vi "Error Converter (ErrCode or Status).vi"(8 "error in (no error)":errorcluster, 11 "error code":i32) -> (0 "error out":errorcluster)   [LabVIEW 2020, in "sqlite3.lvlib"]
uses:
  sqlite3.lvlib
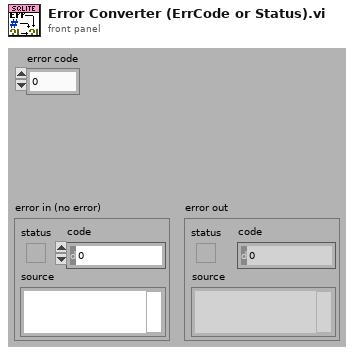
[diagram p1: front panel]
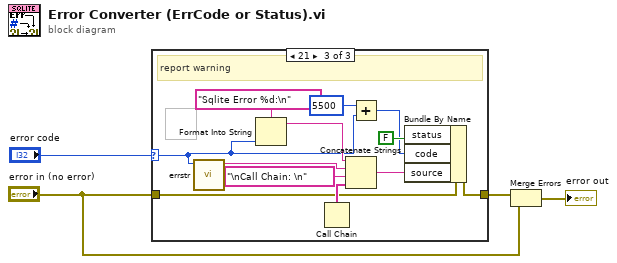
[diagram p0: block diagram]
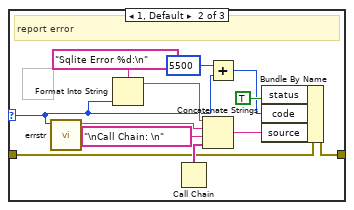
[diagram p3: hidden frame]
diagram:
  n1 = case shown="21" "error code" {
    selector: "error code" -> [_ w7 w19]
    tunnel: [w5 w13 w25] -> w4
    tunnel: "error in (no error)" -> [w5 w14 w26]
    frame 0, 100, 101 {
      # "0 - ok\n100 - more rows\n101 - done"
      # "Not errors"
    }
    frame 1, Default {
      # "report error"
      n2 = call "errstr.vi"("para0"=w7) -> ("function return"=w17:string)  [unwired: 9 in, 1 out]
      n3 = Format Into String(format string="Sqlite Error %d:\n" ("string"), w7) -> (resulting string=w9:string)  [unwired: 2 in, 1 out]
      n4 = Call Chain() -> (call chain=w15:string[])
      n5 = Concatenate Strings(w9, w17, "\nCall Chain: \n" ("string"), w15) -> (w12:string)
      n6 = Add(x=5500, y=w7) -> (x+y=w6:i32)
      n7 = Bundle By Name(cluster=w14, "status"=TRUE ("show call chain? (False)"), "code"=w6, "source"=w12) -> (w13:errorcluster)
    }
    frame 21 {
      # "report warning"
      n8 = call "errstr.vi"("para0"=w19) -> ("function return"=w29:string)  [unwired: 9 in, 1 out]
      n9 = Format Into String(format string="Sqlite Error %d:\n" ("string"), w19) -> (resulting string=w21:string)  [unwired: 2 in, 1 out]
      n10 = Call Chain() -> (call chain=w27:string[])
      n11 = Concatenate Strings(w21, w29, "\nCall Chain: \n" ("string"), w27) -> (w24:string)
      n12 = Add(x=5500, y=w19) -> (x+y=w18:i32)
      n13 = Bundle By Name(cluster=w26, "status"=FALSE ("show call chain? (False)"), "code"=w18, "source"=w24) -> (w25:errorcluster)
    }
  }
  n14 = Merge Errors(w4, "error in (no error)") -> (→"error out":errorcluster)
